vi "daq.vi"() -> ()   [LabVIEW 2015]
uses:
  <vilib>/Instr/_visa.llb/VISA Configure Serial Port (Instr).vi
  <vilib>/Utility/file.llb/Write Delimited Spreadsheet (string).vi
panel:
  in  "Sample Name":string
  out "Flux 2":dbl caption="Volume (mL)" format="%.2g"
  out "rt-weight":dbl
  out "RT wt.":dbl caption="Weight (g)" format="%.1f"
  in  "Pressure Sampling Delay (ms)":u16(knob)=10 max=5000 step=10 scale=10.0..5000.0
  out "Inlet Pressure":dbl caption="Inlet Pressure (psi)" format="%.1f"
  out "Average Flux":dbl(graph)
  out "Average Pressure":dbl(graph)
  in  "Sampling Avg. Lengths":u16=25
  out "Status:":bool caption="2017-05-25 3:51 PM\n0 min"
  in  "Debug":bool=TRUE
  out "Aquired Data (Real Time)":cluster{"Scalar":dbl, "Filtered Volume":dbl}(graph)
  in  "Stop":bool
  out "Flux":dbl caption="Flux (mL/s)" format="%.1f"
  in  "Save Path":path
  in  "Data Preview":i32(listbox)
  in  "Flux Avg. Length":u16=25
  in  "Membrane Area":dbl=1.0
  in  "USB DAQ":tag="cDAQ2Mod1"
  in  "Filtrate Density":dbl=1.0
  in  "Flag":bool=TRUE
  in  "Balance":refnum<visa-resource-name>="COM5"
  # "Liquid-Gated Membrane"
  # "Real-Time Data Acquisition System"
  # "Setup"
  # "Measurement Settings"
  # "Experimental Parameters"
  # "Flux"
  # "Pressure"
  # "Started:"
  # "Elapsed Time:"
  # "COM Settings"
  # "Last Updated: May 2017 • Chris Williams"
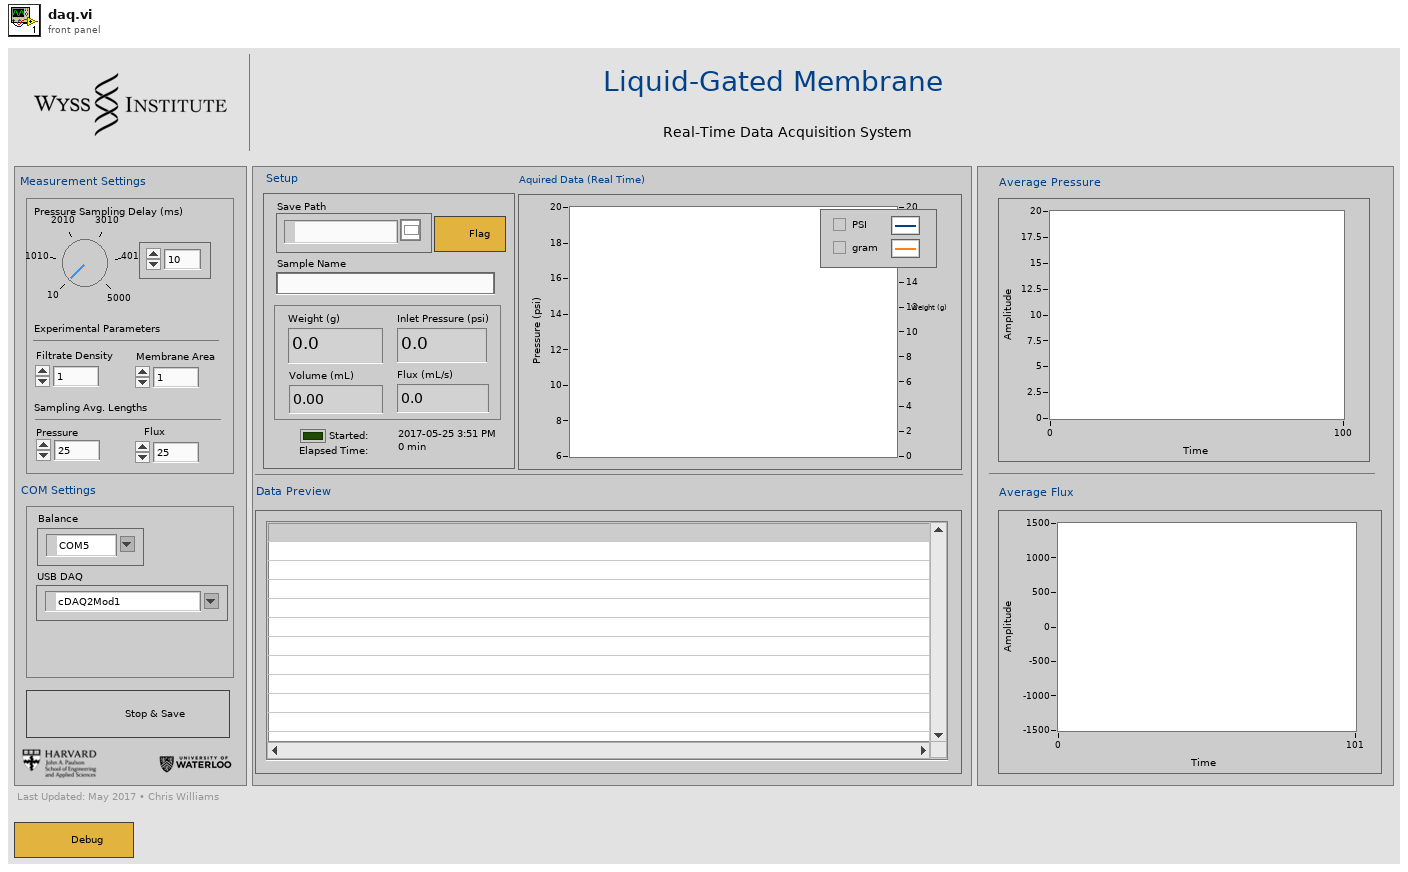
[diagram p1: front panel]
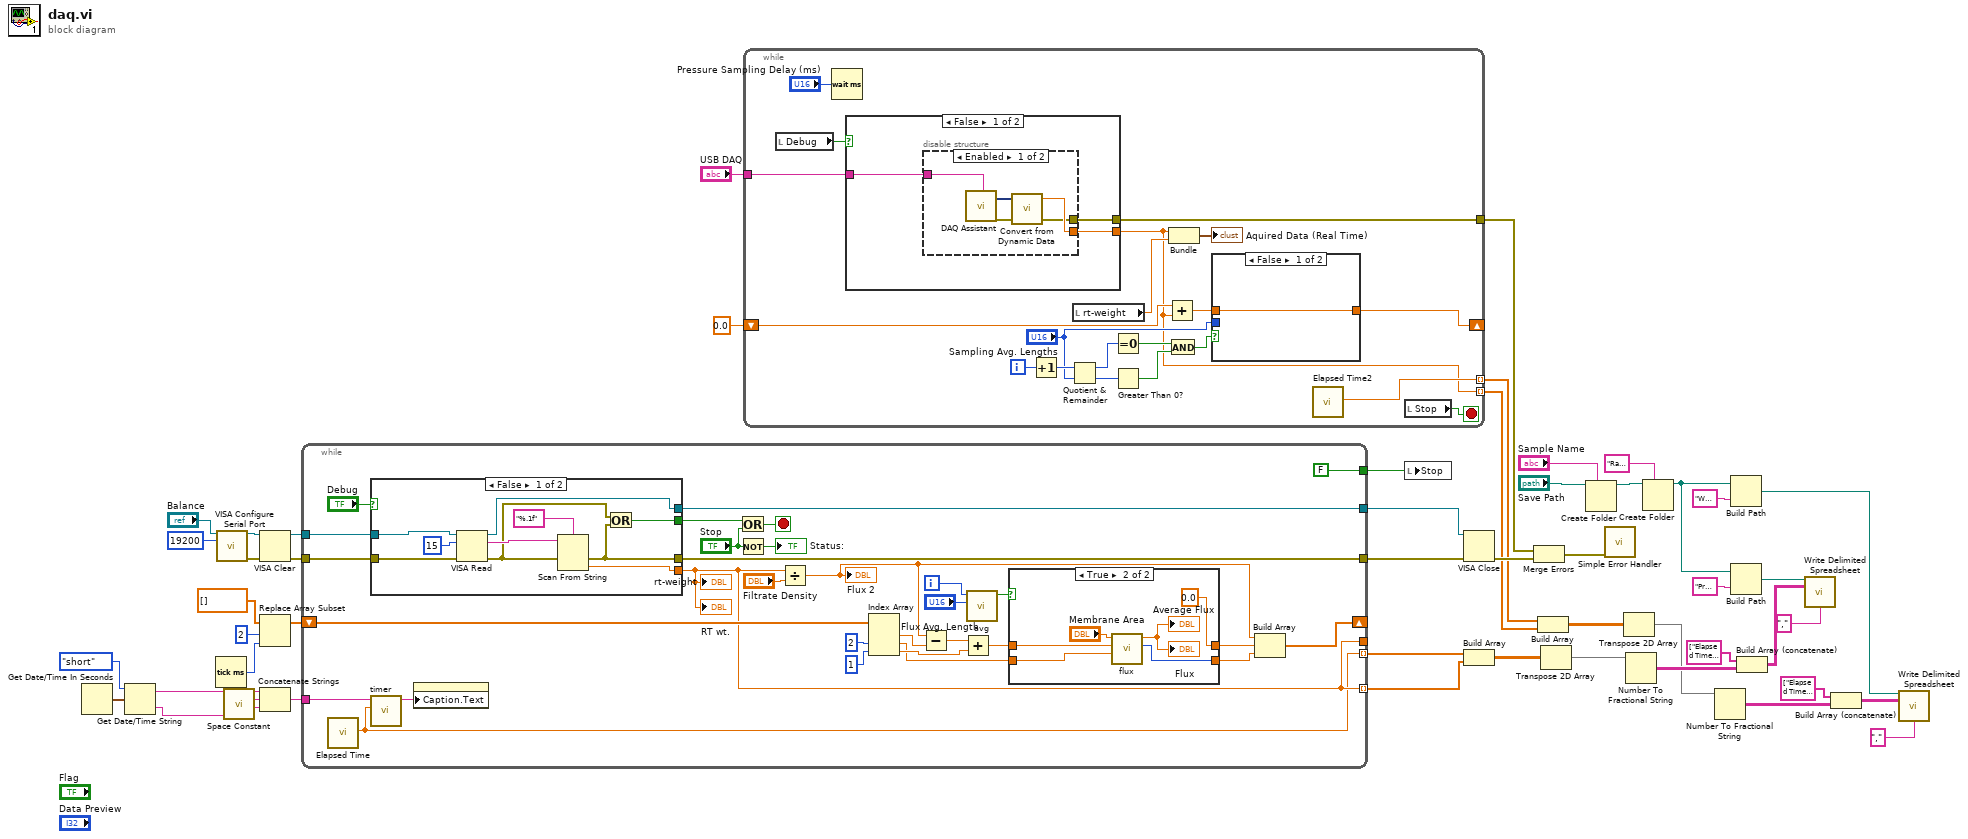
[diagram p0: block diagram]
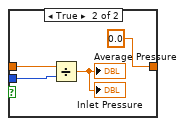
[diagram p2: hidden frame]
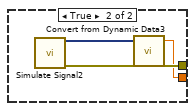
[diagram p4: hidden frame]
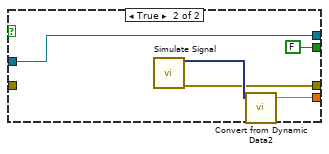
[diagram p6: hidden frame]
diagram:
  n1 = Get Date/Time In Seconds() -> (seconds since 1Jan1904=w36:timestamp)
  n2 = Get Date/Time String(date format (0)=enum16{"short", "long", "abbreviated"}."short", seconds (now)=w36) -> (date string=w33:string, time string=w32:string)  [unwired: 1 in]
  n3 = Tick Count (ms)() -> (millisecond timer value=w28:u32)
  n4 = call-poly "VISA Configure Serial Port"("VISA resource name"="Balance", "baud rate (9600)"=u32 19200) -> ("VISA resource name out"=w45:refnum<visa-resource-name>, "error out"=w43:errorcluster)  [unwired: 12 in]
  n5 = call <vilib>:"Space Constant.vi"() -> ("String"=w34:string)
  n6 = VISA Clear(VISA resource name=w45, error in (no error)=w43) -> (VISA resource name out=w44:refnum<visa-resource-name>, error out=w42:errorcluster)
  n7 = Replace Array Subset(array=dbl[] [], new element=w28, index=2) -> (w27:dbl[])
  n8 = Concatenate Strings(w33, w34, w32) -> (w14:string)
  n9 = while {
    tunnel: w42 -> [w75]
    tunnel: [w76] -> w47
    tunnel: w44 -> [w77]
    tunnel: [w79] -> w46
    shift-right: [w53] -> _
    shift-left: w27 -> [w62]
    tunnel: [FALSE ("Stop")] -> w31
    tunnel: [w52] -> _
    tunnel: [w52] -> w25 mode=indexing
    tunnel: [w51] -> w26 mode=indexing
    tunnel: w14 -> [w50]
    i -> [w72]
    stop <- w69 stop-if-true
    n10 = call "Elapsed Time"() -> ("Elapsed Time (s)"=w51:dbl)  [unwired: 12 in, 7 out]
    n11 = case shown="False" "Debug" {
      tunnel: [w97 w99] -> w79
      tunnel: [w94 w101] -> w52
      tunnel: w75 -> [w93 _]
      tunnel: w77 -> [w92 w99]
      tunnel: [w88 w100] -> w76
      tunnel: [w90 FALSE] -> w74
      frame False {
        n12 = VISA Read(VISA resource name=w92, byte count=u32 15, error in (no error)=w93) -> (VISA resource name out=w97:refnum<visa-resource-name>, read buffer=w96:string, error out=w89:errorcluster)  [unwired: 1 out]
        n13 = Scan From String(format string="%.1f", input string=w96, error in=w89) -> (error out=w88:errorcluster, output 1=w94:dbl)  [unwired: 2 in, 2 out]
        n14 = Or(x=w89, y=w88) -> (x .or. y?=w90:bool)
      }
      frame True {
        n15 = call "Simulate Signal"() -> ("Triangle"=w102:dynamicdata, "error out"=w100:errorcluster)  [unwired: 14 in]
        n16 = call "Convert from Dynamic Data2"("Dynamic Data Type"=w102) -> ("Scalar"=w101:dbl)  [unwired: 3 in]
      }
    }
    "rt-weight" <- w52
    "RT wt." <- w52
    n17 = call "timer.vi"("Elapsed Time (s)"=w51, "string"=w50) -> ("String"=w66:string)  [unwired: 9 in]
    n18 = property on="Status:" class="Bool (strict)"("Caption.Text"=w66) -> ()  [unwired: 2 in, 2 out]
    n19 = Or(x=w74, y="Stop") -> (x .or. y?=w69:bool)
    n20 = Not(x="Stop") -> (.not. x?=→"Status:":bool)
    n21 = Divide(x=w52, y="Filtrate Density") -> (x/y=w56:dbl)
    "Flux 2" <- w56
    n22 = Index Array(array=w62, index #2=2 ("index"), index #3=1 ("index")) -> (element #1=w59:dbl, element #2=w57:dbl, element #3=w58:dbl)  [unwired: 1 in]
    n23 = Subtract(x=w56, y=w59) -> (x-y=w64:dbl)
    n24 = Add(x=w64, y=w58) -> (x+y=w71:dbl)
    n25 = call "avg.vi"("Flux Avg. Length"="Flux Avg. Length", "Numeric"=w72) -> ("Boolean"=w63:bool)  [unwired: 9 in]
    n26 = case shown="True" w63 {
      tunnel: w71 -> [w81 w86]
      tunnel: [w81 0.0 ("x+y")] -> w55
      tunnel: [w80 w83] -> w54
      tunnel: w57 -> [w80 w84]
      frame False {
      }
      frame True {
        n27 = call "flux.vi"("millisecond timer value in"=w84, "Numeric in"=w86, "Membrane Area"="Membrane Area") -> ("millisecond timer value out"=w83:u32, "Numeric out"=→"Average Flux" →"Flux":dbl)  [unwired: 7 in]
      }
    }
    n28 = Build Array(w56, w55, w54) -> (w53:dbl[])
  }
  n29 = while {
    tunnel: "USB DAQ" -> [w122]
    tunnel: [w121] -> w41
    shift-right: [w116] -> _
    shift-left: 0.0 ("Scalar") -> [w118]
    tunnel: [w104] -> w12 mode=indexing
    tunnel: [w103] -> w11 mode=indexing
    i -> [w115]
    stop <- w120 stop-if-true
    n30 = local read "Debug"() -> (w119:bool)
    n31 = Wait (ms)(milliseconds to wait="Pressure Sampling Delay (ms)") -> ()  [unwired: 1 out]
    n32 = case shown="False" w119 {
      tunnel: w122 -> [w130 _]
      tunnel: [w129 w137] -> w121
      tunnel: [w128 w135] -> w103
      frame False {
        n33 = disable-structure shown="Enabled" {
          disable-tunnel: w130 -> [w134 _]
          disable-tunnel: [w131 _] -> w129
          disable-tunnel: [w132 _] -> w128
          frame Enabled {
            n34 = call "DAQ Assistant"("device name"=w134) -> ("data"=w133:dynamicdata, "error out"=w131:errorcluster)  [unwired: 15 in, 2 out]
            n35 = call "Convert from Dynamic Data"("Dynamic Data Type"=w133) -> ("Scalar"=w132:dbl)  [unwired: 3 in]
          }
          frame Disabled {
          }
        }
      }
      frame True {
        n36 = call "Simulate Signal2"() -> ("Sine with Uniform Noise"=w136:dynamicdata, "error out"=w137:errorcluster)  [unwired: 14 in]
        n37 = call "Convert from Dynamic Data3"("Dynamic Data Type"=w136) -> ("Scalar"=w135:dbl)  [unwired: 3 in]
      }
    }
    n38 = Increment(x=w115) -> (x+1=w114:i32)
    n39 = Quotient & Remainder(x=w114, y="Sampling Avg. Lengths") -> (x-y*floor(x/y)=w113:i32, floor(x/y)=w112:i32)
    n40 = local read "rt-weight"() -> (w106:dbl)
    n41 = Equal To 0?(x=w113) -> (x = 0?=w111:bool)
    n42 = Greater Than 0?(x=w112) -> (x > 0?=w110:bool)
    n43 = Add(x=w118, y=w103) -> (x+y=w117:dbl)
    n44 = And(x=w111, y=w110) -> (x .and. y?=w109:bool)
    n45 = Bundle("Scalar"=w103, "rt-weight"=w106) -> (→"Aquired Data (Real Time)":cluster{"Scalar":dbl, "rt-weight":dbl})  [unwired: 1 in]
    n46 = case shown="False" w109 {
      tunnel: w117 -> [w123 w127]
      tunnel: [w123 0.0] -> w116
      tunnel: "Sampling Avg. Lengths" -> [_ w126]
      frame False {
      }
      frame True {
        n47 = Divide(x=w127, y=w126) -> (x/y=→"Average Pressure" →"Inlet Pressure":dbl)
      }
    }
    n48 = call "Elapsed Time2"() -> ("Elapsed Time (s)"=w104:dbl)  [unwired: 12 in, 7 out]
    n49 = local read "Stop"() -> (w120:bool)
  }
  n50 = local write "Stop"(w31) -> ()
  n51 = VISA Close(VISA resource name=w46, error in (no error)=w47) -> (error out=w40:errorcluster)
  n52 = Build Array(w26, w25) -> (w24:dbl[][])
  n53 = Merge Errors(w41, w40) -> (w39:errorcluster)
  n54 = Build Array(w12, w11) -> (w10:dbl[][])
  n55 = Transpose 2D Array(2D array=w24) -> (transposed array=w18:dbl[][])
  n56 = Create Folder(prompt (Create Folder)="Sample Name", path (use dialog)="Save Path") -> (created path=w16:path)  [unwired: 1 in, 2 out]
  n57 = call <vilib>:"Simple Error Handler.vi"("error in (no error)"=w39) -> ()  [unwired: 4 in, 5 out]
  n58 = Transpose 2D Array(2D array=w10) -> (transposed array=w5:dbl[][])
  n59 = Number To Fractional String(number=w18) -> (F-format string=w23:string[][])  [unwired: 3 in]
  n60 = Create Folder(prompt (Create Folder)="Raw Data", path (use dialog)=w16) -> (created path=w4:path)  [unwired: 1 in, 2 out]
  n61 = Number To Fractional String(number=w5) -> (F-format string=w9:string[][])  [unwired: 3 in]
  n62 = Build Path(base path=w4, name or relative path="Weight.csv") -> (appended path=w2:path)
  n63 = Build Path(base path=w4, name or relative path="Pressure.csv" ("string")) -> (appended path=w19:path)
  n64 = Build Array (concatenate)(string[] ["Elapsed Time (s)", "Pressure (PSIG)"], w23) -> (w21:string[][])
  n65 = call-poly <vilib>:"Write Delimited Spreadsheet.vi"("file path (dialog if empty)"=w19, "2D data"=w21, "delimiter (\\t)"="," ("delimiter (\\t)")) -> ()  [unwired: 11 in, 2 out]
  n66 = Build Array (concatenate)(string[] ["Elapsed Time (s)", "Weight (g)"], w9) -> (w7:string[][])
  n67 = call-poly <vilib>:"Write Delimited Spreadsheet.vi"("file path (dialog if empty)"=w2, "2D data"=w7, "delimiter (\\t)"="," ("delimiter (\\t)")) -> ()  [unwired: 11 in, 2 out]
